vi "PH_Switch.check 6P Switch.vi"(0 "Tagname":string) -> (1 "Tagname 6P Switch":string, 2 "6P Switch?":bool)   [LabVIEW 2014, in "PH_Switch.lvlib"]
doc: "This VI checks wether \"6P::\" is part of the name of the Tag. If so, and if the string behind is not empty, this is given out as \"Tagname 6P Switch\" (N/A otherwise), and \"6P Switch?\" is true."
uses:
  PH_Switch.lvlib
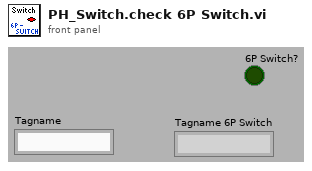
[diagram p1: front panel]
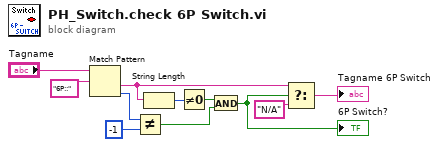
[diagram p0: block diagram]
diagram:
  n1 = Match Pattern(string="Tagname", regular expression="6P::") -> (after substring=w5:string, offset past match=w9:i32)  [unwired: 1 in, 2 out]
  n2 = Not Equal?(x=w9, y=-1) -> (x != y?=w2:bool)
  n3 = String Length(string=w5) -> (length=w4:i32)
  n4 = Not Equal To 0?(x=w4) -> (x != 0?=w3:bool)
  n5 = And(x=w3, y=w2) -> (x .and. y?=w1:bool)
  "6P Switch?" <- w1
  n6 = Select(t=w5, s=w1, f="N/A") -> (s? t:f=→"Tagname 6P Switch":string)
